vi "Post-Init.vi"(8 "error in (no error)":errorcluster, 11 "Instrument Driver in":refnum<class "Instrument Driver.lvclass">) -> (0 "error out":errorcluster, 2 "Init Result":refnum<class "Acquired Result.lvclass">, 3 "Instrument Driver out":refnum<class "Instrument Driver.lvclass">)   [LabVIEW 2015, in "Instrument Driver.lvclass"]
uses:
  Instrument Driver.lvclass
  Measure_core/Results/Acquired Result/Acquired Result.lvclass
  Instrument Driver.lvclass/Instrument Driver.ctl
  Measure_core/Results/Acquired Result/Acquired Result.lvclass/Acquired Result.ctl
  Read Group name.vi
  Read Channel names.vi
  Measure_core/Results/Acquired Result/Write Group.vi
  Measure_core/Results/Acquired Result/Write Channels.vi
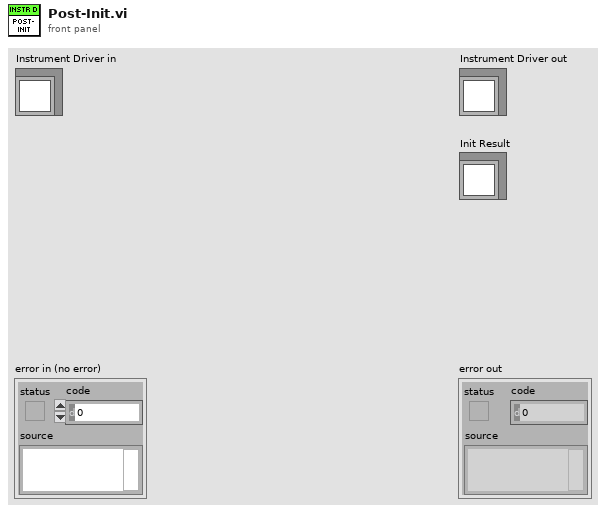
[diagram p1: front panel]
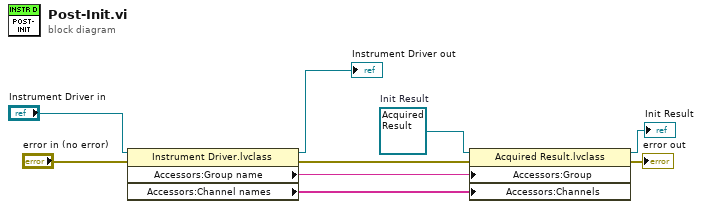
[diagram p0: block diagram]
diagram:
  w8 = refnum<class "Acquired Result.lvclass"> refnum  # Init Result
  n1 = property class="Instrument Driver.lvclass"(reference="Instrument Driver in", error in="error in (no error)") -> (reference out=→"Instrument Driver out":refnum<class "Instrument Driver.lvclass">, error out=w4:errorcluster, "Accessors:Group name"=w5:string, "Accessors:Channel names"=w1:string[])
  n2 = property class="Acquired Result.lvclass"(reference=w8, error in=w4, "Accessors:Group"=w5, "Accessors:Channels"=w1) -> (reference out=→"Init Result":refnum<class "Acquired Result.lvclass">, error out=→"error out":errorcluster)
